vi "Stop Core.vi"(10 "final error code":i32, 11 "Instrument Handler in":refnum<class "Instrument Handler.lvclass">) -> (3 "Instrument Handler out":refnum<class "Instrument Handler.lvclass">)   [LabVIEW 2020, in "Instrument Handler.lvlib" / "Instrument Handler.lvclass"]
doc: "(<B>Filename</B>: Actor Framework.lvlib:Actor.lvclass:Stop Core.vi)\n\nDefines what the actor does before it stops. Use the <B>final error code</B> input to determine whether the actor shut down in response to an error.\n\nThis implementation initiates the shut down of all owned processes."
uses:
  Instrument Handler.lvclass
  Controls/Ctl_InstrumentSynchronicationCluster.ctl
  PPL/HDH.Actor Framework.Core.Instrument Driver.lvlibp/Instrument Driver/Controls/Ctl_ConnectionType.ctl
  PPL/HDH.Data.Generic.lvlibp/Synchronization/Notifier/Notifier.lvclass
  PPL/HDH.Actor Framework.Core.Actor.lvlibp/1abvi3w/vi.lib/ActorFramework/Message Enqueuer/Message Enqueuer.lvclass
  PPL/HDH.Actor Framework.Core.Sequencer.lvlibp/Sequencer Core/Sequencer Core.lvclass
  Instrument Handler.lvclass/Instrument Handler.ctl
  Enqueuer Global.vi
  PPL/HDH.Actor Framework.Core.Actor.lvlibp/1abvi3w/vi.lib/ActorFramework/Actor/Actor.lvclass
  PPL/HDH.Actor Framework.Core.Instrument Driver.lvlibp/Instrument Driver/Instrument Driver.lvclass
  Instrument Handler.lvlib
  PPL/HDH.Actor Framework.Core.Actor.lvlibp/1abvi3w/vi.lib/ActorFramework/Stop Msg/Stop Msg.lvclass
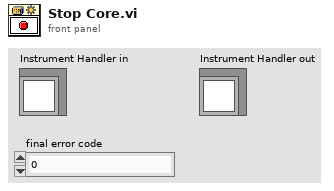
[diagram p1: front panel]
types:
  T1 = typedef "Semaphore RefNum" = refnum<k1>
  T2 = typedef "Instrument Handler.lvlib/Ctl_AquirerAvailabilityStatus.ctl" = cluster{"Available?":bool, "Aquirer":T3}
  T3 = typedef "Instrument Handler.lvlib/Ctl_AquirerRefnum.ctl" = refnum<vi>
  T4 = typedef "Instrument Handler.lvlib/Ctl_InstrumentSynchronicationCluster.ctl" = cluster{"Launched?":bool, "Driver Path":path, "Alias":string, "Connection Type":T5, "Pre Initialization Data":variant, "Enqueue Sync":refnum<class "Notifier.lvclass">, "Enqueue Lock":T1, "Owner Enqueuer":refnum<class "Message Enqueuer.lvclass">, "Owner":refnum<class "Sequencer Core.lvclass">, "Instrument ID":u32}
  T5 = typedef "HDH.Actor Framework.Core.Instrument Driver.lvlibp/Instrument Driver.lvclass/Ctl_ConnectionType.ctl" = enum16{"BuiltIn/System", "PXI/PCI", "USB", "GPIB", "VXI", "Serial", "TCP/IP", "cRIO", "SCXI", "cDAQ", "SwitchBlock", "SCC", "FireWire", "Accessory", "CAN", "SwitchBlock Device"}
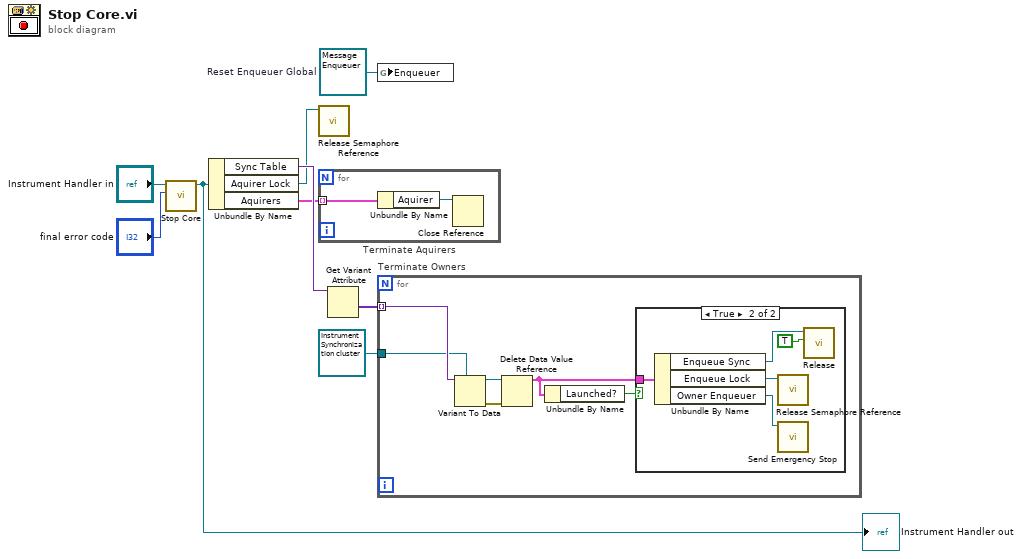
[diagram p0: block diagram]
diagram:
  w1 = refnum<class "Message Enqueuer.lvclass"> refnum  # Reset Enqueuer Global
  n1 = call-parent "Stop Core.vi"("final error code"="final error code", "Actor in"="Instrument Handler in") -> ("Actor out"=w7:refnum<class "Instrument Handler.lvclass">)  [unwired: 9 in]
  "Instrument Handler out" <- w7
  n2 = Unbundle By Name(w7) -> ("Sync Table"=w6:variant, "Aquirer Lock"=w3:T1, "Aquirers"=w2:T2[])
  n3 = call <vilib>:"Release Semaphore Reference.vi"("semaphore"=w3) -> ()  [unwired: 9 in, 2 out]
  n4 = for "Terminate Aquirers" {
    tunnel: w2 -> [w11] mode=indexing
    n5 = Unbundle By Name(w11) -> ("Aquirer"=w10:T3)
    n6 = Close Reference(reference=w10) -> ()  [unwired: 1 in, 1 out]
  }
  n7 = Get Variant Attribute(Variant=w6) -> (values=w5:variant[])  [unwired: 3 in, 3 out]
  n8 = global write "Enqueuer Global.vi" "Enqueuer"(w1) -> ()
  n9 = for "Terminate Owners" {
    tunnel: w5 -> [w17] mode=indexing
    tunnel: refnum<data-value> refnum ("data value reference") -> [w16]
    n10 = Variant To Data(type=w16, Variant=w17) -> (data=w15:refnum<data-value>, error out=w14:errorcluster)  [unwired: 1 in]
    n11 = Delete Data Value Reference(data value reference=w15, error in=w14) -> (data value=w12:T4)  [unwired: 1 out]
    n12 = Unbundle By Name(w12) -> ("Launched?"=w13:bool)
    n13 = case shown="True" w13 {
      tunnel: w12 -> [_ w22]
      frame False {
      }
      frame True {
        n14 = Unbundle By Name(w22) -> ("Enqueue Sync"=w20:refnum<class "Notifier.lvclass">, "Enqueue Lock"=w21:T1, "Owner Enqueuer"=w18:refnum<class "Message Enqueuer.lvclass">)
        n15 = call <vilib>:"Release Semaphore Reference.vi"("semaphore"=w21) -> ()  [unwired: 9 in, 2 out]
        n16 = call "Send Emergency Stop.vi"("Message Enqueuer"=w18) -> ()  [unwired: 10 in, 1 out]
        n17 = call "Release.vi"("Force destroy? (F)"=TRUE, "Notifier in"=w20) -> ()  [unwired: 7 in, 3 out]
      }
    }
  }
